vi "Car Wash Server.vi"() -> ()   [LabVIEW 2024]
uses:
  Control 3.ctl
  <vilib>/Utility/file.llb/Read Delimited Spreadsheet (string).vi
  <vilib>/Utility/file.llb/Write Delimited Spreadsheet (string).vi
  <vilib>/regexp/Match Regular Expression.xnode
panel:
  in  "Tab Control":T1(tab)
  in  "Login Button":bool
  in  "Admin Password":string
  in  "Admin Username":string
  out "Log Table":string[][](table)
  in  "Log Back Button":bool
  in  "View User Button":bool
  in  "View Data Button":bool
  in  "Choose Function Back Button":bool
  out "User Table":string[][](table)
  in  "User Back Button":bool
  out "error out":errorcluster
  # "Wash Log"
  # "User Credentials"
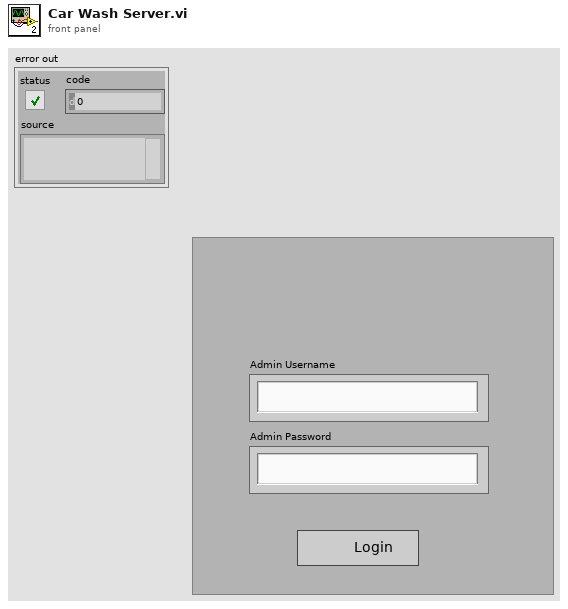
[diagram p1: front panel]
types:
  T1 = enum32{"Login Page", "Log Page", "Selection Page", "User Credential Page"}
  T2 = typedef "Control 3.ctl" = enum16{"Init", "Login", "View Data", "View User Credentials", "Select Funciton"}
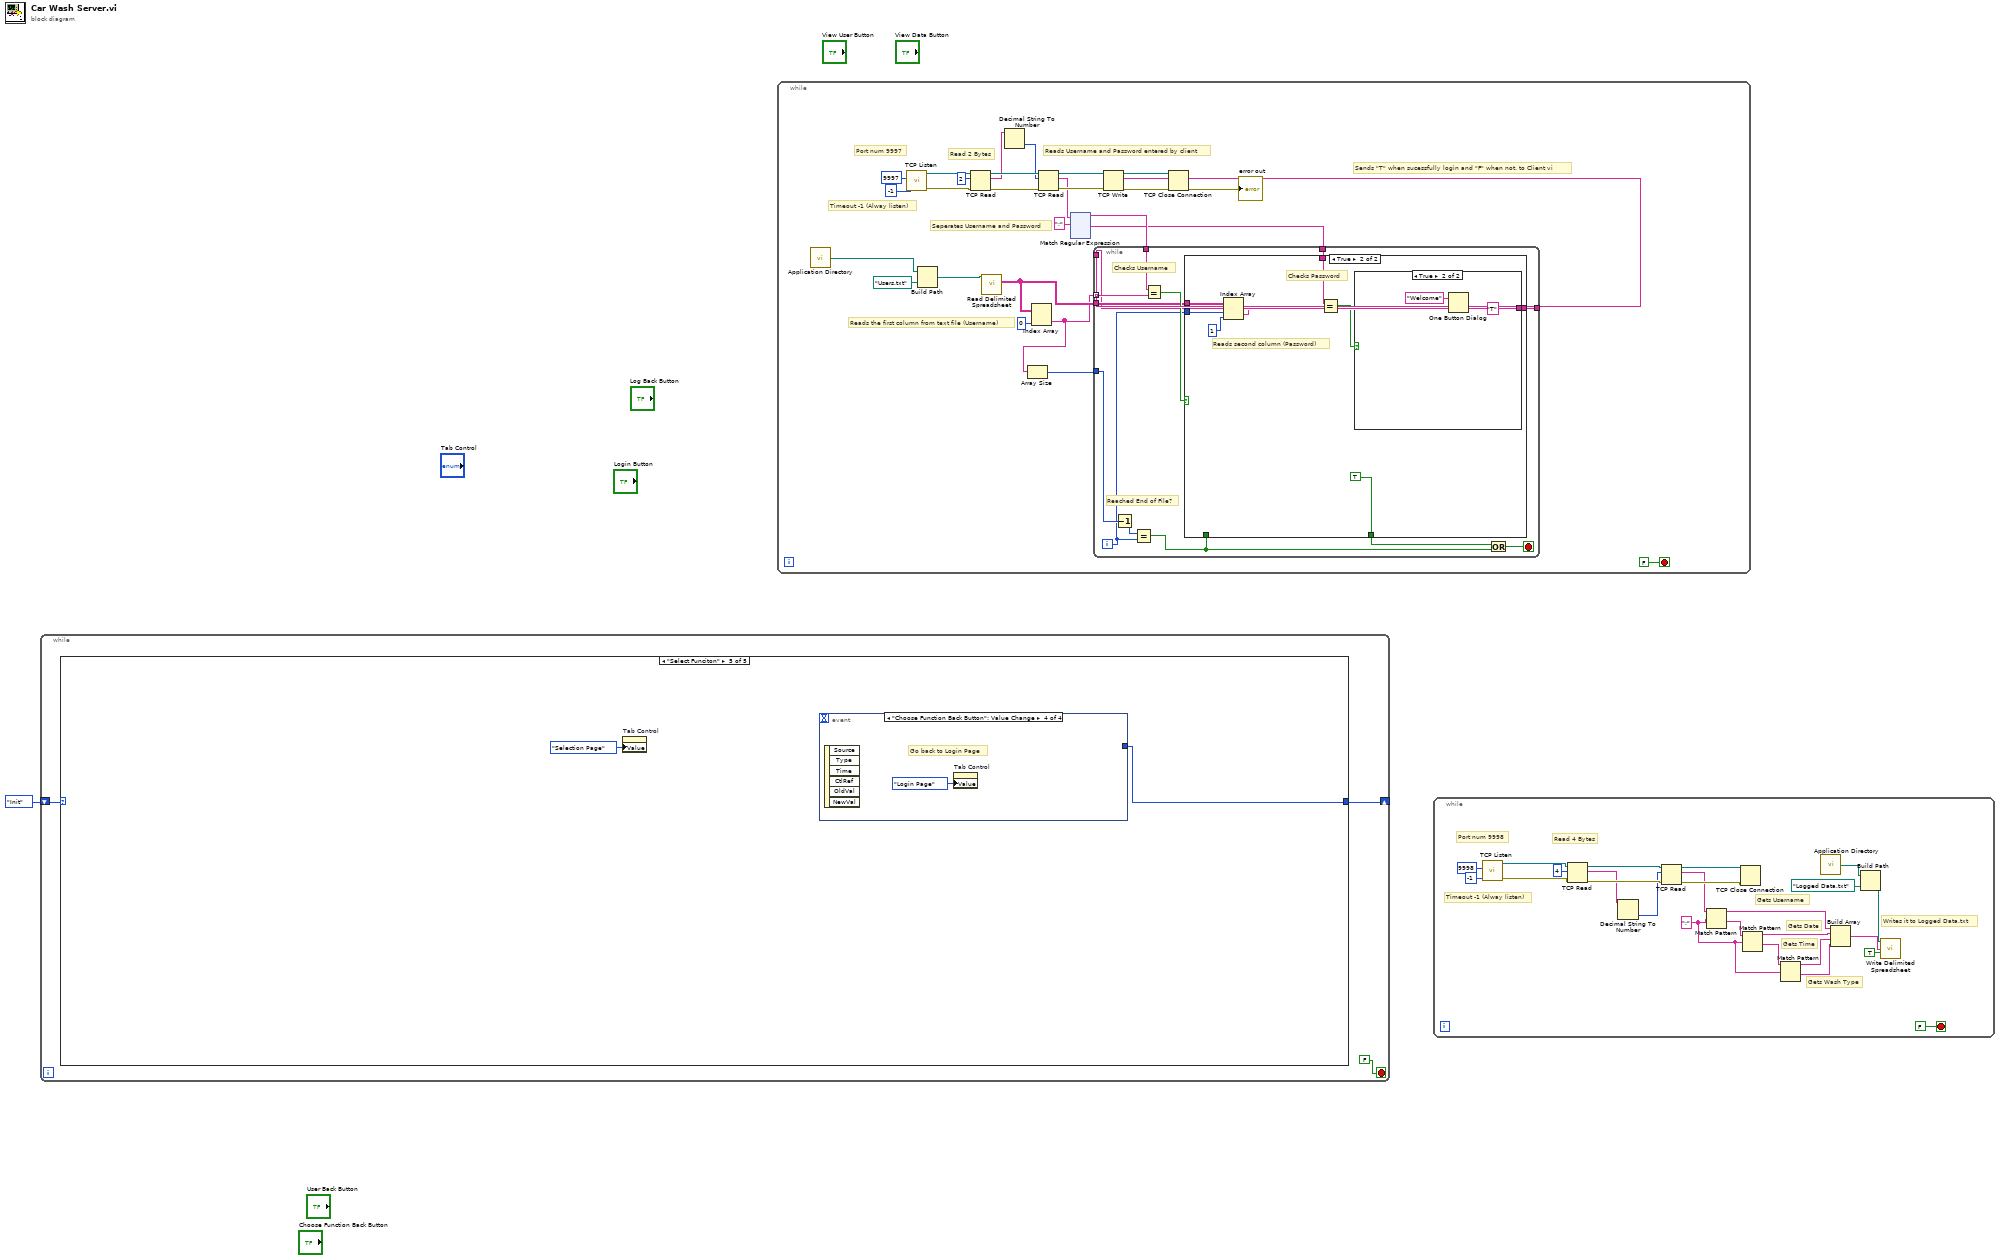
[diagram p0: block diagram]
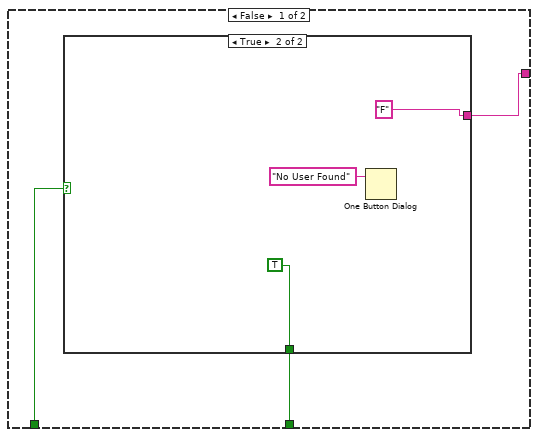
[diagram p2: hidden frame]
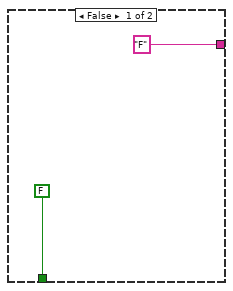
[diagram p3: hidden frame]
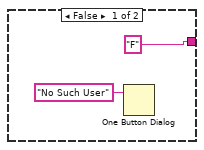
[diagram p4: hidden frame]
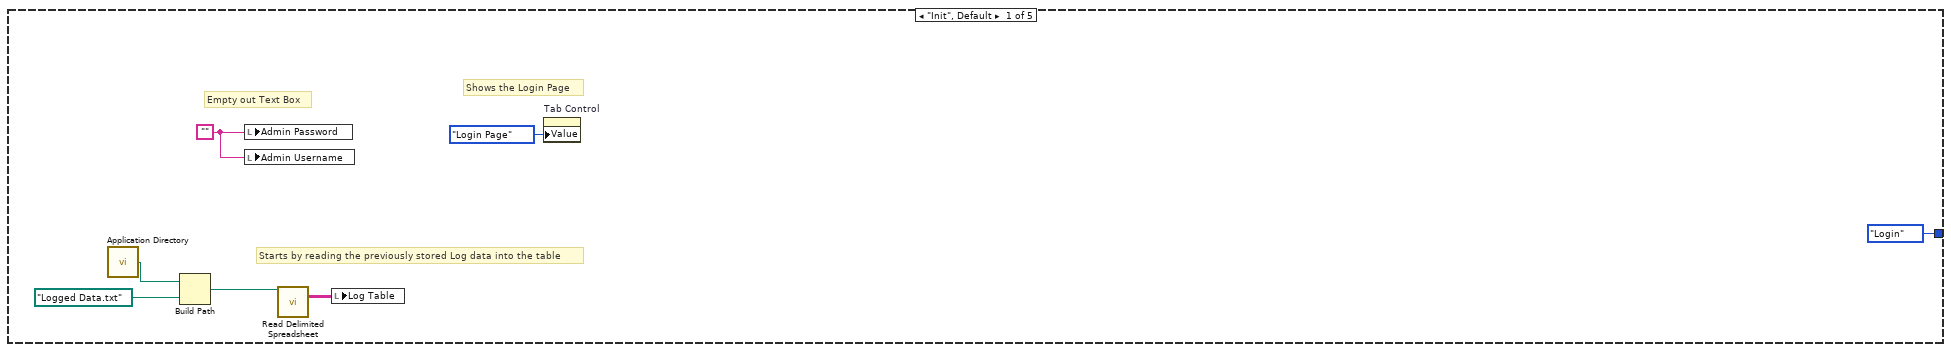
[diagram p5: hidden frame]
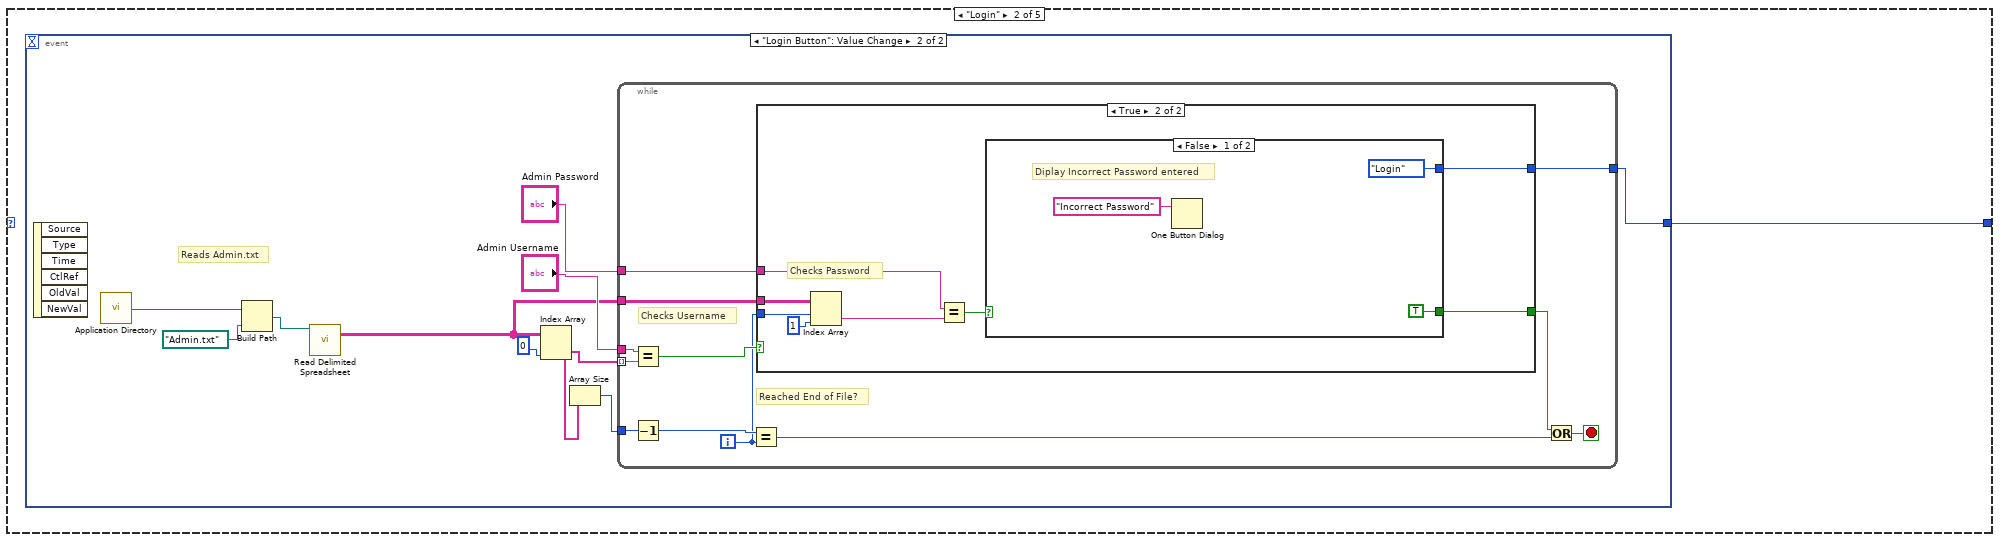
[diagram p6: hidden frame]
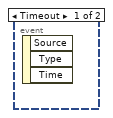
[diagram p7: hidden frame]
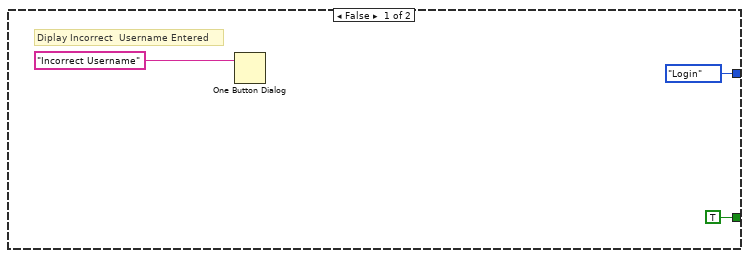
[diagram p8: hidden frame]
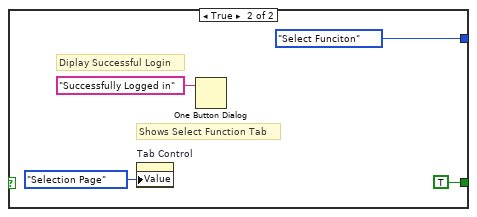
[diagram p9: hidden frame]
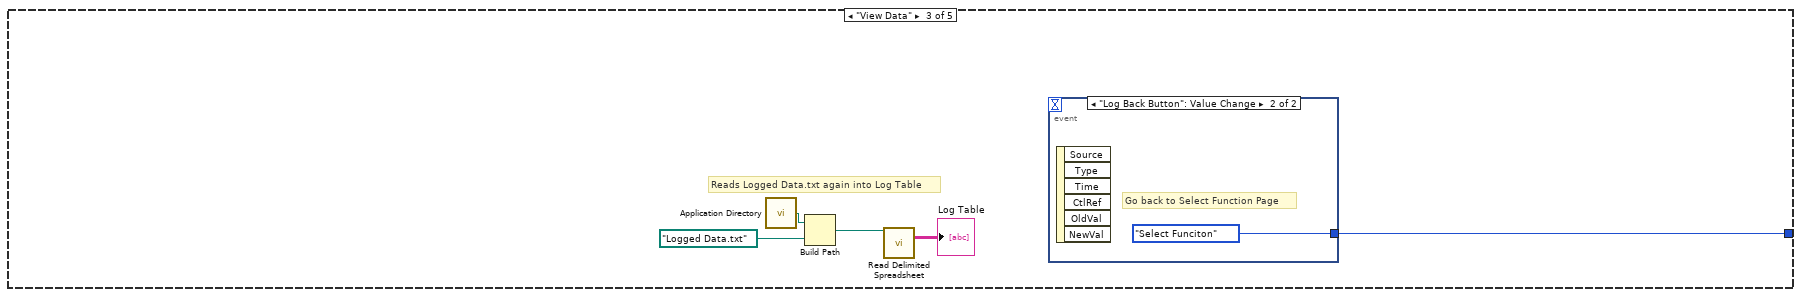
[diagram p10: hidden frame]
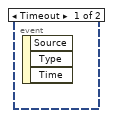
[diagram p11: hidden frame]
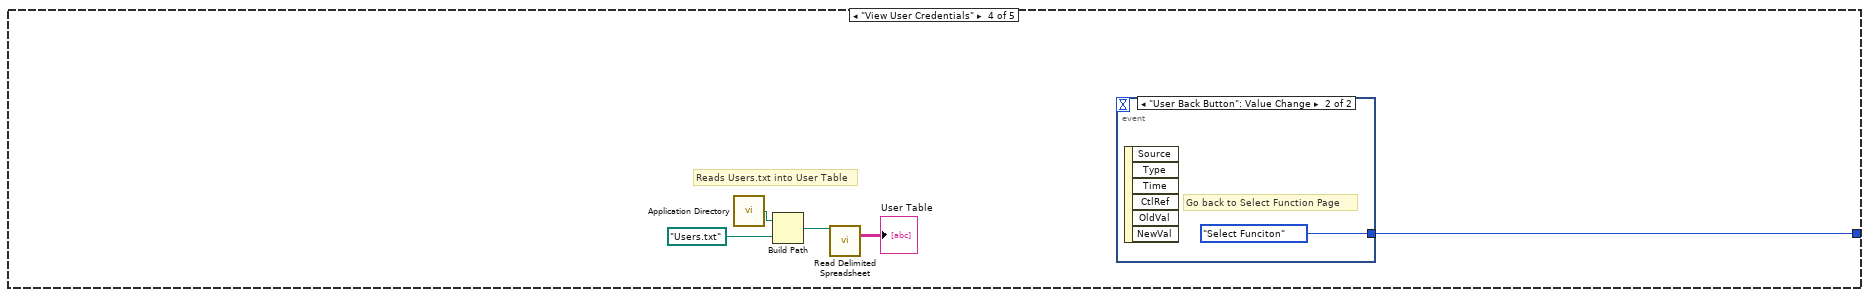
[diagram p12: hidden frame]
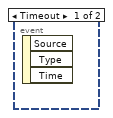
[diagram p13: hidden frame]
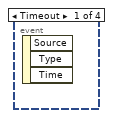
[diagram p14: hidden frame]
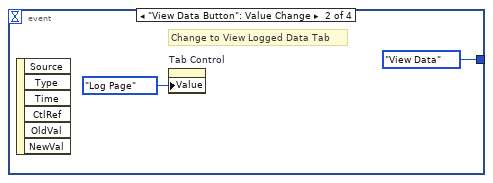
[diagram p15: hidden frame]
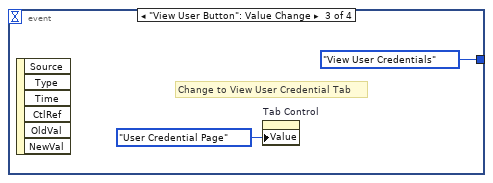
[diagram p16: hidden frame]
diagram:
  n1 = while {
    shift-right: [w2] -> _
    shift-left: Control_3."Init" -> [w3]
    stop <- FALSE stop-if-true
    n2 = case shown="\"Select Funciton\"" w3 {
      tunnel: [Control_3."Login" w12 w53 w59 w66] -> w2
      frame "Init", Default {
        w11 = ""
        # "Empty out Text Box"
        # "Shows the Login Page"
        # "Starts by reading the previously stored Log data into the table"
        n3 = call <vilib>:"Application Directory.vi"() -> ("Application Directory"=w8:path)
        n4 = Build Path(base path=w8, name or relative path=path "Logged Data.txt") -> (appended path=w9:path)
        n5 = local write "Admin Password"(w11) -> ()
        n6 = local write "Admin Username"(w11) -> ()
        n7 = call-poly <vilib>:"Read Delimited Spreadsheet.vi"("file path (dialog if empty)"=w9) -> ("all rows"=w6:string[][])  [unwired: 9 in, 5 out]
        n8 = local write "Log Table"(w6) -> ()
        n9 = property on="Tab Control" class="TabCtl (strict)"("Value"=T1."Login Page" ("Tab Control")) -> ()  [unwired: 2 in, 2 out]
      }
      frame "Login" {
        n10 = event shown="[1] \"Login Button\": Value Change" {
          selector: _ -> [_ _]
          dyn-events: _ -> [_ _]
          timeout: _ -> [_ _]
          tunnel: [_ w14] -> w12
          event Timeout {
            n11 = event-data() -> ()  [unwired: 1 in, 3 out]
          }
          event "Login Button": Value Change {
            # "Reads Admin.txt"
            n12 = event-data() -> ()  [unwired: 1 in, 6 out]
            n13 = call <vilib>:"Application Directory.vi"() -> ("Application Directory"=w21:path)
            n14 = Build Path(base path=w21, name or relative path=path "Admin.txt") -> (appended path=w22:path)
            n15 = call-poly <vilib>:"Read Delimited Spreadsheet.vi"("file path (dialog if empty)"=w22) -> ("all rows"=w18:string[][])  [unwired: 9 in, 5 out]
            n16 = Index Array "Index Array"(array=w18, index (col)=0 ("disabled index (col)")) -> (element=w17:string[])  [unwired: 1 in]
            n17 = Array Size(array=w17) -> (size(s)=w16:i32)
            n18 = while {
              tunnel: "Admin Username" -> [w34]
              tunnel: w17 -> [w33] mode=indexing
              tunnel: w18 -> [w31]
              tunnel: w16 -> [w30]
              tunnel: "Admin Password" -> [w27]
              tunnel: [w26] -> w14
              i -> [w28]
              stop <- w23 stop-if-true
              # "Reached End of File?"
              # "Checks Username"
              n19 = Equal?(x=w34, y=w33) -> (x = y?=w32:bool)
              n20 = Decrement(x=w30) -> (x-1=w29:i32)
              n21 = Equal?(x=w29, y=w28) -> (x = y?=w25:bool)
              n22 = case shown="True" w32 {
                tunnel: w31 -> [_ w45]
                tunnel: w28 -> [_ w43]
                tunnel: w27 -> [_ w42]
                tunnel: [Control_3."Login" w39] -> w26
                tunnel: [TRUE w38] -> w24
                frame False {
                  # "Diplay Incorrect  Username Entered"
                  n23 = One Button Dialog(message="Incorrect Username") -> ()  [unwired: 1 in, 1 out]
                }
                frame True {
                  # "Checks Password"
                  n24 = Index Array(array=w45, index (row)=w43, index (col)=1 ("disabled index (col)")) -> (element=w41:string)
                  n25 = Equal?(x=w42, y=w41) -> (x = y?=w40:bool)
                  n26 = case shown="False" w40 {
                    tunnel: [Control_3."Login" Control_3."Select Funciton"] -> w39
                    tunnel: [TRUE TRUE] -> w38
                    frame False {
                      # "Diplay Incorrect Password entered"
                      n27 = One Button Dialog(message="Incorrect Password") -> ()  [unwired: 1 in, 1 out]
                    }
                    frame True {
                      # "Diplay Successful Login"
                      # "Shows Select Function Tab"
                      n28 = property on="Tab Control" class="TabCtl (strict)"("Value"=T1."Selection Page" ("Tab Control")) -> ()  [unwired: 2 in, 2 out]
                      n29 = One Button Dialog(message="Successfully Logged in") -> ()  [unwired: 1 in, 1 out]
                    }
                  }
                }
              }
              n30 = Or(x=w24, y=w25) -> (x .or. y?=w23:bool)
            }
          }
        }
      }
      frame "View Data" {
        # "Reads Logged Data.txt again into Log Table"
        n31 = call <vilib>:"Application Directory.vi"() -> ("Application Directory"=w55:path)
        n32 = Build Path(base path=w55, name or relative path=path "Logged Data.txt") -> (appended path=w56:path)
        n33 = call-poly <vilib>:"Read Delimited Spreadsheet.vi"("file path (dialog if empty)"=w56) -> ("all rows"=→"Log Table":string[][])  [unwired: 9 in, 5 out]
        n34 = event shown="[1] \"Log Back Button\": Value Change" {
          selector: _ -> [_ _]
          dyn-events: _ -> [_ _]
          timeout: _ -> [_ _]
          tunnel: [_ Control_3."Select Funciton"] -> w53
          event Timeout {
            n35 = event-data() -> ()  [unwired: 1 in, 3 out]
          }
          event "Log Back Button": Value Change {
            # "Go back to Select Function Page"
            n36 = event-data() -> ()  [unwired: 1 in, 6 out]
          }
        }
      }
      frame "View User Credentials" {
        # "Reads Users.txt into User Table"
        n37 = call <vilib>:"Application Directory.vi"() -> ("Application Directory"=w63:path)
        n38 = Build Path(base path=w63, name or relative path=path "Users.txt") -> (appended path=w61:path)
        n39 = call-poly <vilib>:"Read Delimited Spreadsheet.vi"("file path (dialog if empty)"=w61) -> ("all rows"=→"User Table":string[][])  [unwired: 9 in, 5 out]
        n40 = event shown="[1] \"User Back Button\": Value Change" {
          selector: _ -> [_ _]
          dyn-events: _ -> [_ _]
          timeout: _ -> [_ _]
          tunnel: [_ Control_3."Select Funciton"] -> w59
          event Timeout {
            n41 = event-data() -> ()  [unwired: 1 in, 3 out]
          }
          event "User Back Button": Value Change {
            # "Go back to Select Function Page"
            n42 = event-data() -> ()  [unwired: 1 in, 6 out]
          }
        }
      }
      frame "Select Funciton" {
        n43 = property on="Tab Control" class="TabCtl (strict)"("Value"=T1."Selection Page" ("Tab Control")) -> ()  [unwired: 2 in, 2 out]
        n44 = event shown="[3] \"Choose Function Back Button\": Value Change" {
          selector: _ -> [_ _ _ _]
          dyn-events: _ -> [_ _ _ _]
          timeout: _ -> [_ _ _ _]
          tunnel: [_ Control_3."View Data" Control_3."View User Credentials" _] -> w66
          event Timeout {
            n45 = event-data() -> ()  [unwired: 1 in, 3 out]
          }
          event "View Data Button": Value Change {
            # "Change to View Logged Data Tab"
            n46 = event-data() -> ()  [unwired: 1 in, 6 out]
            n47 = property on="Tab Control" class="TabCtl (strict)"("Value"=T1."Log Page" ("Tab Control")) -> ()  [unwired: 2 in, 2 out]
          }
          event "View User Button": Value Change {
            # "Change to View User Credential Tab"
            n48 = event-data() -> ()  [unwired: 1 in, 6 out]
            n49 = property on="Tab Control" class="TabCtl (strict)"("Value"=T1."User Credential Page" ("Tab Control")) -> ()  [unwired: 2 in, 2 out]
          }
          event "Choose Function Back Button": Value Change {
            # "Go back to Login Page"
            n50 = event-data() -> ()  [unwired: 1 in, 6 out]
            n51 = property on="Tab Control" class="TabCtl (strict)"("Value"=T1."Login Page" ("Tab Control")) -> ()  [unwired: 2 in, 2 out]
          }
        }
      }
    }
  }
  n52 = while {
    stop <- FALSE stop-if-true
    # "Sends \"T\" when sucessfully login and \"F\" when not, to Client vi"
    # "Timeout -1 (Alway listen)"
    # "Port num 9997"
    # "Read 2 Bytes"
    # "Reads the first column from text file (Username)"
    # "Seperates Username and Password"
    # "Reads Username and Password entered by client"
    n53 = call <vilib>:"Application Directory.vi"() -> ("Application Directory"=w75:path)
    n54 = call <vilib>:"TCP Listen.vi"("timeout ms (wait forever: -1)"=-1, "port"=u16 9997) -> ("error out"=w94:errorcluster, "connection ID"=w98:refnum<k5>)  [unwired: 5 in, 3 out]
    n55 = Build Path(base path=w75, name or relative path=path "Users.txt") -> (appended path=w76:path)
    n56 = TCP Read(connection ID=w98, bytes to read=2, error in (no error)=w94) -> (connection ID out=w97:refnum<k5>, data out=w87:string, error out=w93:errorcluster)  [unwired: 2 in]
    n57 = call-poly <vilib>:"Read Delimited Spreadsheet.vi"("file path (dialog if empty)"=w76) -> ("all rows"=w83:string[][])  [unwired: 9 in, 5 out]
    n58 = Decimal String To Number(string=w87) -> (number=w86:i32)  [unwired: 2 in, 1 out]
    n59 = Index Array "Index Array"(array=w83, index (col)=0 ("disabled index (col)")) -> (element=w81:string[])  [unwired: 1 in]
    n60 = Array Size(array=w81) -> (size(s)=w82:i32)
    n61 = TCP Read(connection ID=w97, bytes to read=w86, error in (no error)=w93) -> (connection ID out=w96:refnum<k5>, data out=w85:string, error out=w92:errorcluster)  [unwired: 2 in]
    n62 = xnode "Match Regular Expression"("input string"=w85, "regular expression"=";") -> ("before match"=w79:string, "after match"=w78:string)  [unwired: 4 in, 3 out]
    n63 = while {
      tunnel: w81 -> [w110] mode=indexing
      tunnel: w82 -> [w106]
      tunnel: w83 -> [w103]
      tunnel: w79 -> [w101]
      tunnel: w78 -> [w100]
      tunnel: [w99] -> _
      tunnel: [w99] -> w77
      i -> [w102]
      stop <- w109 stop-if-true
      # "Reached End of File?"
      # "Checks Username"
      n64 = Decrement(x=w106) -> (x-1=w107:i32)
      n65 = Equal?(x=w107, y=w102) -> (x = y?=w105:bool)
      n66 = Equal?(x=w101, y=w110) -> (x = y?=w108:bool)
      n67 = case shown="True" w108 {
        tunnel: [w113 TRUE] -> w104
        tunnel: w105 -> [w112 _]
        tunnel: w103 -> [_ w122]
        tunnel: w102 -> [_ w121]
        tunnel: w100 -> [_ w120]
        tunnel: [w111 w119] -> w99
        frame False {
          n68 = case shown="True" w112 {
            tunnel: [FALSE TRUE] -> w113
            tunnel: ["F" "F"] -> w111
            frame False {
            }
            frame True {
              n69 = One Button Dialog(message="No User Found") -> ()  [unwired: 1 in, 1 out]
            }
          }
        }
        frame True {
          # "Reads second column (Password)"
          # "Checks Password"
          n70 = Index Array "Index Array"(array=w122, index (row)=w121, index (col)=1 ("disabled index (col)")) -> (element=w125:string)
          n71 = Equal?(x=w120, y=w125) -> (x = y?=w124:bool)
          n72 = case shown="True" w124 {
            tunnel: ["F" "T"] -> w119
            frame False {
              n73 = One Button Dialog(message="No Such User") -> ()  [unwired: 1 in, 1 out]
            }
            frame True {
              n74 = One Button Dialog(message="Welcome") -> ()  [unwired: 1 in, 1 out]
            }
          }
        }
      }
      n75 = Or(x=w104, y=w105) -> (x .or. y?=w109:bool)
    }
    n76 = TCP Write(connection ID=w96, data in=w77, error in (no error)=w92) -> (connection ID out=w95:refnum<k5>, error out=w91:errorcluster)  [unwired: 1 in, 1 out]
    n77 = TCP Close Connection(connection ID=w95, error in (no error)=w91) -> (error out=→"error out":errorcluster)  [unwired: 1 in, 1 out]
  }
  n78 = while {
    stop <- FALSE stop-if-true
    w249 = ";" ("regular expression")
    # "Writes it to Logged Data.txt"
    # "Gets Time"
    # "Gets Wash Type"
    # "Gets Date"
    # "Gets Username"
    # "Read 4 Bytes"
    # "Timeout -1 (Alway listen)"
    # "Port num 9998"
    n79 = call <vilib>:"TCP Listen.vi"("timeout ms (wait forever: -1)"=-1, "port"=u16 9998) -> ("error out"=w267:errorcluster, "connection ID"=w270:refnum<k5>)  [unwired: 5 in, 3 out]
    n80 = TCP Read(connection ID=w270, bytes to read=4, error in (no error)=w267) -> (connection ID out=w269:refnum<k5>, data out=w263:string, error out=w266:errorcluster)  [unwired: 2 in]
    n81 = Decimal String To Number(string=w263) -> (number=w262:i32)  [unwired: 2 in, 1 out]
    n82 = TCP Read(connection ID=w269, bytes to read=w262, error in (no error)=w266) -> (connection ID out=w268:refnum<k5>, data out=w257:string, error out=w265:errorcluster)  [unwired: 2 in]
    n83 = Match Pattern(string=w257, regular expression=w249) -> (before substring=w255:string, after substring=w256:string)  [unwired: 1 in, 2 out]
    n84 = TCP Close Connection(connection ID=w268, error in (no error)=w265) -> ()  [unwired: 1 in, 2 out]
    n85 = Match Pattern(string=w256, regular expression=w249) -> (before substring=w254:string, after substring=w253:string)  [unwired: 1 in, 2 out]
    n86 = Match Pattern(string=w253, regular expression=w249) -> (before substring=w252:string, after substring=w251:string)  [unwired: 1 in, 2 out]
    n87 = call <vilib>:"Application Directory.vi"() -> ("Application Directory"=w261:path)
    n88 = Build Array "Build Array"(w255, w254, w252, w251) -> (w250:string[])
    n89 = Build Path(base path=w261, name or relative path=path "Logged Data.txt") -> (appended path=w259:path)
    n90 = call-poly <vilib>:"Write Delimited Spreadsheet.vi"("file path (dialog if empty)"=w259, "1D data"=w250, "append to file? (new file:F)"=TRUE) -> ()  [unwired: 11 in, 2 out]
  }
